vi "Read Drive Base Operation.vi"(8 "Command Info":T3) -> (0 "Command Info":T3, 1 "SubSystem Data":T1, 2 "Command Timing":cluster{"Start Time (ms)":u32, "Iterations":i32})   [LabVIEW 2019]
doc: "This returns the most recently scheduled command. This doesn't indicate whether the command finished and is running the default command."
uses:
  <vilib>/Rock Robotics/WPI/Framework/Command Status Info.ctl
  <vilib>/Rock Robotics/WPI/Framework/Completion Status.ctl
  <vilib>/Rock Robotics/WPI/Framework/Completion Notifier.ctl
  Implementation/Drive Base Setpoints.ctl
  Implementation/Drive Base Operations.ctl
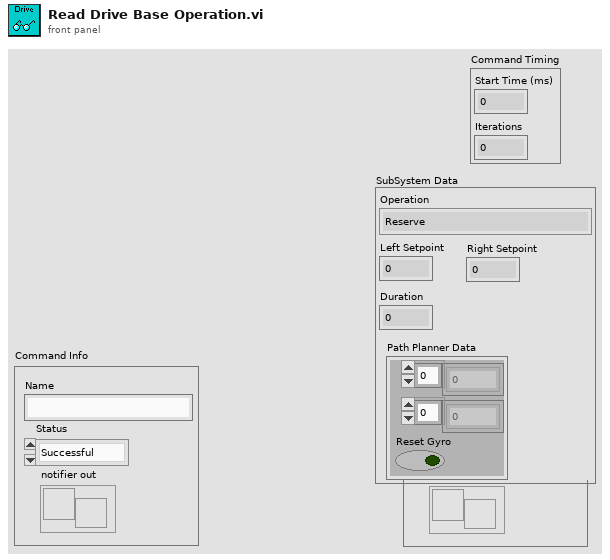
[diagram p1: front panel]
types:
  T1 = typedef "Drive Base Setpoints.ctl" = cluster{"Operation":T2, "Left Setpoint":dbl, "Duration":dbl, "Right Setpoint":dbl, "Path Planner Data":cluster{dbl[], dbl[], "Reset Gyro":bool}}
  T2 = typedef "Drive Base Operations.ctl" = enum16{"Reserve", "Read Current", "Immediate", "Limelight", "Manual Adjustment", "Play Path"}
  T3 = typedef "Command Status Info.ctl" = cluster{"Name":string, "Status":T4, "notifier out":T5}
  T4 = typedef "Completion Status.ctl" = enum16{"Successful", "Aborted", "Incomplete"}
  T5 = typedef "Completion Notifier.ctl" = refnum<notifier>
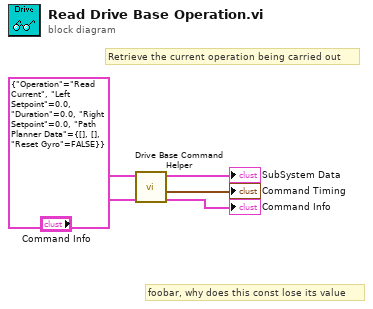
[diagram p0: block diagram]
diagram:
  # "foobar, why does this const lose its value"
  # "Retrieve the current operation being carried out"
  n1 = call "Drive Base Command Helper.vi"("Command Info In"="Command Info", "SubSystem Data"=T1 {"Operation"=enum."Read Current", "Left Setpoint"=0.0, "Duration"=0.0, "Right Setpoint"=0.0, "Path Planner Data"={[], [], "Reset Gyro"=FALSE}}) -> ("Command Info Out"=→"Command Info":T3, "Command Timing"=→"Command Timing":cluster{"Start Time (ms)":u32, "Iterations":i32}, "SubSystem Data"=→"SubSystem Data":T1)  [unwired: 7 in]
